vi "boolean.vi"() -> ()   [LabVIEW 2018]
panel:
  in  "?":bool
  out "Boolean 18":bool
  out "Boolean 17":bool
  out "Boolean 16":bool
  out "Boolean 15":bool
  out "Boolean 14":bool
  out "Boolean 13":bool
  in  "Latch Until Released":bool
  in  "Latch When Released":bool
  in  "Latch When Pressed":bool
  in  "Switch Until Released":bool
  in  "Switch When Released":bool
  in  "Switch When Pressed":bool
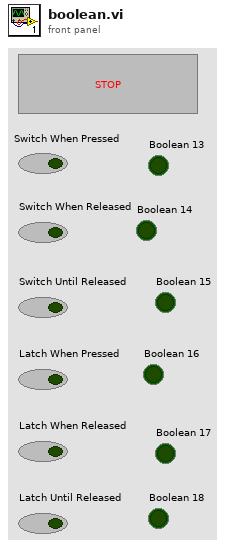
[diagram p1: front panel]
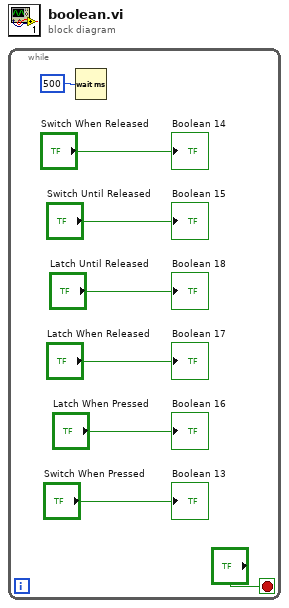
[diagram p0: block diagram]
diagram:
  n1 = while {
    stop <- "?" stop-if-true
    n2 = Wait (ms)(milliseconds to wait=u32 500) -> ()  [unwired: 1 out]
    "Boolean 13" <- "Switch When Pressed"
    "Boolean 14" <- "Switch When Released"
    "Boolean 15" <- "Switch Until Released"
    "Boolean 16" <- "Latch When Pressed"
    "Boolean 17" <- "Latch When Released"
    "Boolean 18" <- "Latch Until Released"
  }
